vi "Set Default Value.vi"(8 "error in (no error)":errorcluster, 10 "Default Value":string, 11 "Sub Object in":refnum<class "Sub Object.lvclass">) -> (0 "error out":errorcluster, 3 "Sub Object out":refnum<class "Sub Object.lvclass">)   [LabVIEW 2019, in "Electronic Datasheet.lvlib" / "Sub Object.lvclass"]
uses:
  Sub Object.lvclass
  Sub Object.lvclass/Sub Object.ctl
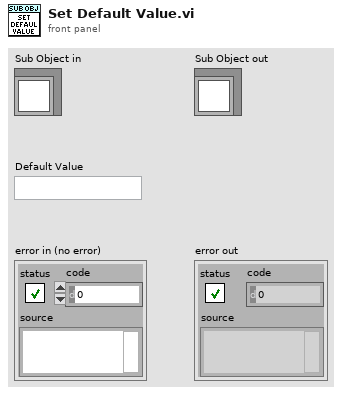
[diagram p1: front panel]
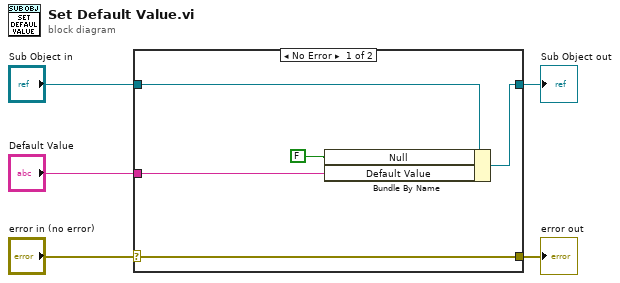
[diagram p0: block diagram]
diagram:
  n1 = case shown="No Error" "error in (no error)" {
    selector: "error in (no error)" -> [w10 w11]
    tunnel: [w10 w11] -> w4
    tunnel: [w8 w12] -> w2
    tunnel: "Sub Object in" -> [w9 w12]
    tunnel: "Default Value" -> [w7 _]
    frame No Error {
      n2 = Bundle By Name(cluster=w9, "Null"=FALSE ("Default Value.Null"), "Default Value"=w7) -> (w8:refnum<class "Sub Object.lvclass">)
    }
    frame Error {
    }
  }
  "error out" <- w4
  "Sub Object out" <- w2
